vi "us open.vi"(8 "error in":errorcluster, 10 "Enum":T1, 11 "my FPGA lib.lvlib:US sensor.lvclass":refnum<class "US sensor.lvclass">) -> (0 "error out":errorcluster, 3 "output cluster":refnum<class "US sensor.lvclass">)   [LabVIEW 2019, in "my FPGA lib.lvlib" / "US sensor.lvclass"]
uses:
  US sensor.lvclass
  us select.ctl
  US sensor.lvclass/US sensor.ctl
  <vilib>/Utility/error.llb/Error Cluster From Error Code.vi
  <vilib>/rvi/errors/niLvFpgaAdjustHostInterfaceError.vi
  <vilib>/rvi/interface/nirviReadWriteControl/nirviReadWriteControl.xnode
  my FPGA lib.lvlib
  <vilib>/rvi/interface/Simulation/niFpgaSimulationCallBeginRW.vi
  NiFpgaLv.dll
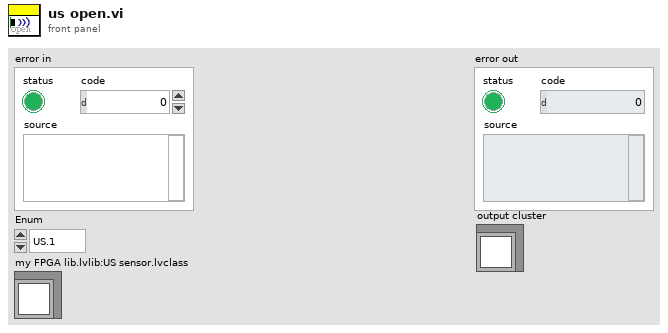
[diagram p1: front panel]
types:
  T1 = typedef "my FPGA lib.lvlib/US sensor.lvclass/us select.ctl" = enum16{"US.1", "US.2", "US.3", "US.4"}
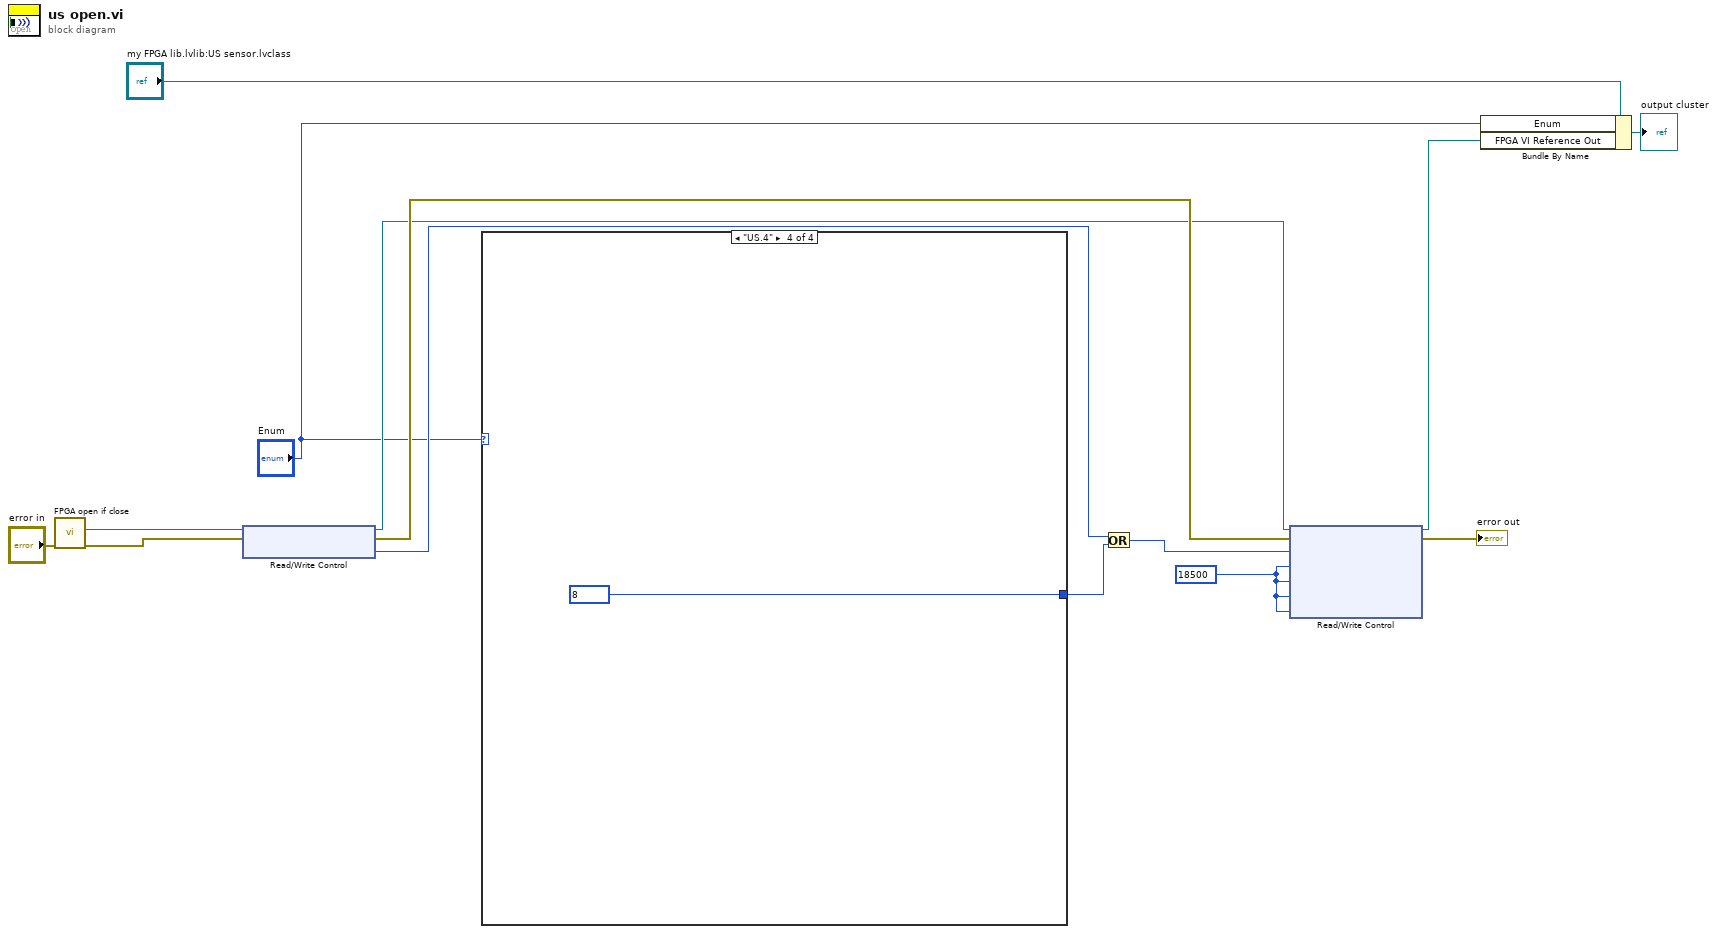
[diagram p0: block diagram]
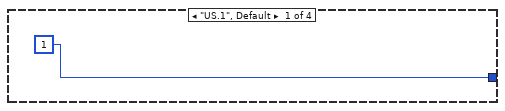
[diagram p2: hidden frame]
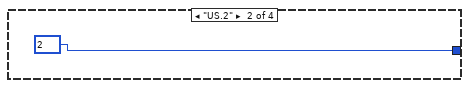
[diagram p3: hidden frame]
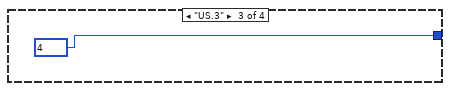
[diagram p4: hidden frame]
diagram:
  w6 = 18500 ("us1.timeout(us)")
  n1 = call "FPGA open if close.vi"("error in"="error in") -> ("error out"=w13:errorcluster, "FPGA VI Reference Out"=w14:refnum<k20>)  [unwired: 9 in]
  n2 = xnode "Read/Write Control"("FPGA VI Reference In"=w14, "error in"=w13) -> ("FPGA VI Reference Out"=w7:refnum<k20>, "error out"=w8:errorcluster, "Ultrasonic.IO.Enable"=w11:u8)
  n3 = case shown="\"US.4\"" "Enum" {
    tunnel: [u8 1 u8 2 u8 4 u8 8] -> w10
    frame "US.1", Default {
    }
    frame "US.2" {
    }
    frame "US.3" {
    }
    frame "US.4" {
    }
  }
  n4 = Or(x=w11, y=w10) -> (x .or. y?=w9:u8)
  n5 = xnode "Read/Write Control"("FPGA VI Reference In"=w7, "error in"=w8, "Ultrasonic.IO.Enable"=w9, "us1.timeout(us)"=w6, "us2.timeout(us)"=w6, "us3.timeout(us)"=w6, "us4.timeout(us)"=w6) -> ("FPGA VI Reference Out"=w2:refnum<k20>, "error out"=→"error out":errorcluster)
  n6 = Bundle By Name(cluster="my FPGA lib.lvlib:US sensor.lvclass", "Enum"="Enum", "FPGA VI Reference Out"=w2) -> (→"output cluster":refnum<class "US sensor.lvclass">)
